vi "IVIS FRET_Load Image Data.vi"(6 "Background File Name":string="luminescent.TIF", 8 "Error In":errorcluster, 9 "# Frames":i32, 10 "Data Folder Root Name":string, 11 "Root Folder":path) -> (0 "Error Out":errorcluster, 1 "[DA Images]":T1[](array[typedef]), 2 "[AA Images]":T1[](array[typedef]), 3 "[DD Images]":T1[](array[typedef]), 4 "Time Stamps":i64[](array[numeric]), 5 "Y Resolution":i32, 7 "X Resolution":i32)   [LabVIEW 2021]
uses:
  <vilib>/vision/Image Controls.llb/IMAQ Image.ctl
  <vilib>/vision/NI_Vision_Development_Module.lvlib
panel:
  out "Same Sizes":bool
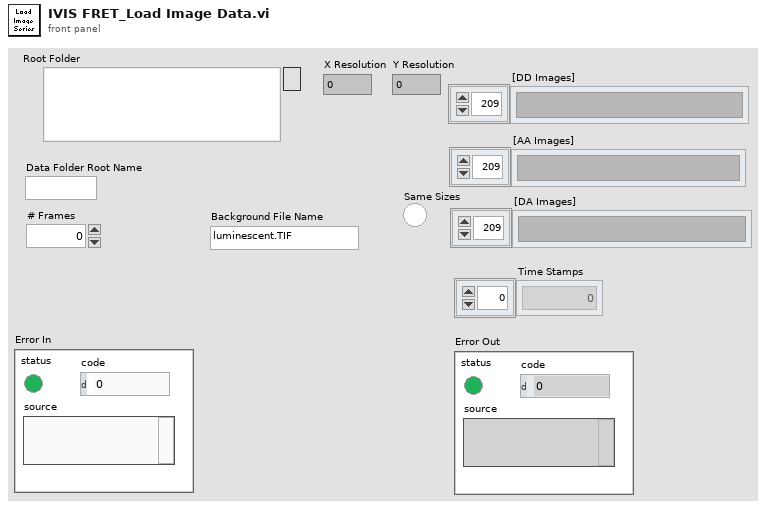
[diagram p1: front panel]
types:
  T1 = typedef "IMAQ Image.ctl" = refnum<image>
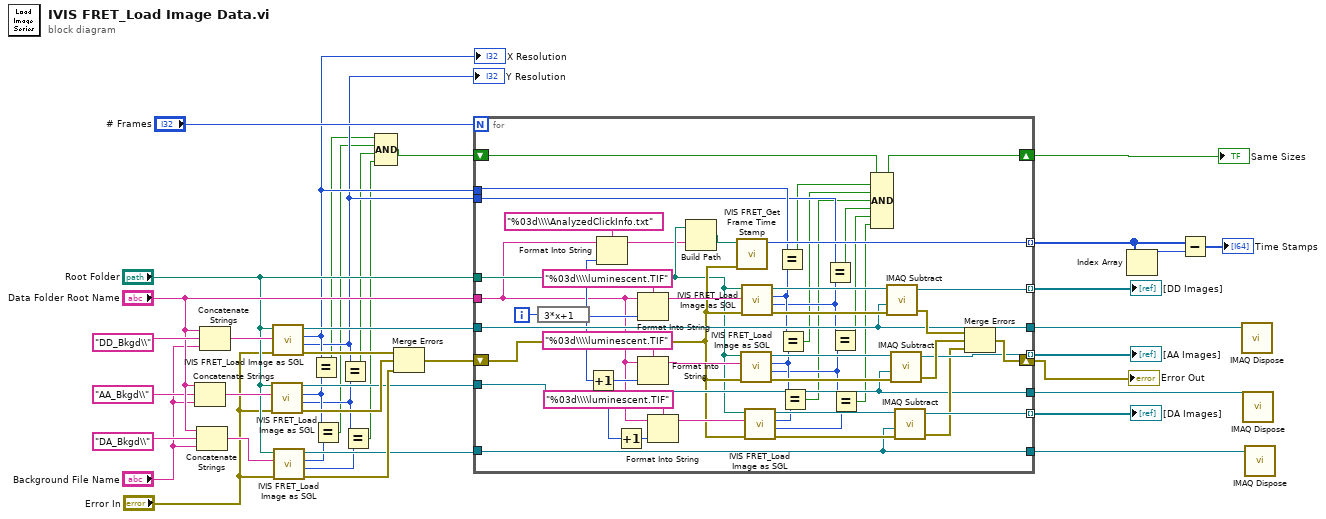
[diagram p0: block diagram]
diagram:
  n1 = Concatenate Strings("Data Folder Root Name", "AA_Bkgd\\" ("format string"), "Background File Name") -> (w27:string)
  n2 = Concatenate Strings("Data Folder Root Name", "DA_Bkgd\\" ("format string"), "Background File Name") -> (w25:string)
  n3 = Concatenate Strings("Data Folder Root Name", "DD_Bkgd\\" ("format string"), "Background File Name") -> (w35:string)
  n4 = call "IVIS FRET_Load Image as SGL.vi"("error in"="Error In", "Image File Name"=w27, "Root Folder"="Root Folder") -> ("error out"=w23:errorcluster, "Y Resolution"=w8:i32, "X Resolution"=w11:i32, "Background Image"=w20:T1)  [unwired: 5 in]
  n5 = call "IVIS FRET_Load Image as SGL.vi"("error in"="Error In", "Image File Name"=w35, "Root Folder"="Root Folder") -> ("error out"=w31:errorcluster, "Y Resolution"=w9:i32, "X Resolution"=w12:i32, "Background Image"=w29:T1)  [unwired: 5 in]
  "X Resolution" <- w12
  "Y Resolution" <- w9
  n6 = call "IVIS FRET_Load Image as SGL.vi"("error in"="Error In", "Image File Name"=w25, "Root Folder"="Root Folder") -> ("error out"=w22:errorcluster, "Y Resolution"=w7:i32, "X Resolution"=w10:i32, "Background Image"=w21:T1)  [unwired: 5 in]
  n7 = Equal?(x=w12, y=w11) -> (x = y?=w6:bool)
  n8 = Equal?(x=w11, y=w10) -> (x = y?=w5:bool)
  n9 = Equal?(x=w9, y=w8) -> (x = y?=w4:bool)
  n10 = Equal?(x=w8, y=w7) -> (x = y?=w3:bool)
  n11 = Compound Arithmetic op=AND(w6, w5, w4, w3) -> (w2:bool)
  n12 = Merge Errors(w31, w23, w22) -> (w28:errorcluster)
  n13 = for {
    N: "# Frames" -> [_]
    tunnel: "Root Folder" -> [w61]
    tunnel: "Data Folder Root Name" -> [w57]
    shift-right: [w86] -> w30
    shift-left: w28 -> [w62]
    tunnel: [w82] -> w39 mode=indexing
    tunnel: [w78] -> w37 mode=indexing
    tunnel: [w79] -> w38 mode=indexing
    tunnel: w29 -> [w70]
    tunnel: w21 -> [w65]
    tunnel: w20 -> [w69]
    tunnel: [w70] -> w19
    tunnel: [w69] -> w18
    tunnel: [w65] -> w17
    tunnel: [w58] -> w15 mode=indexing
    tunnel: w12 -> [w56]
    tunnel: w9 -> [w52]
    shift-right: [w41] -> w1
    shift-left: w2 -> [w42]
    i -> [w88]
    n14 = expression code="3*x+1"(w88) -> (w64:i32)
    n15 = Increment(x=w64) -> (x+1=w83:i32)
    n16 = Format Into String(format string="%03d\\\\AnalyzedClickInfo.txt", initial string=w57, w64) -> (resulting string=w60:string)  [unwired: 1 in, 1 out]
    n17 = Increment(x=w83) -> (x+1=w85:i32)
    n18 = Format Into String(format string="%03d\\\\luminescent.TIF", initial string=w57, w64) -> (resulting string=w68:string)  [unwired: 1 in, 1 out]
    n19 = Format Into String(format string="%03d\\\\luminescent.TIF", initial string=w57, w83) -> (resulting string=w67:string)  [unwired: 1 in, 1 out]
    n20 = Format Into String(format string="%03d\\\\luminescent.TIF", initial string=w57, w85) -> (resulting string=w66:string)  [unwired: 1 in, 1 out]
    n21 = Build Path(base path=w61, name or relative path=w60) -> (appended path=w59:path)
    n22 = call "IVIS FRET_Get Frame Time Stamp.vi"("error in (no error)"=w62, "File Path"=w59) -> ("Time Stamp"=w58:i64)  [unwired: 8 in, 1 out]
    n23 = call "IVIS FRET_Load Image as SGL.vi"("error in"=w62, "Image File Name"=w67, "Root Folder"=w61) -> ("error out"=w73:errorcluster, "Y Resolution"=w49:i32, "X Resolution"=w54:i32, "Background Image"=w74:T1)  [unwired: 5 in]
    n24 = call "IVIS FRET_Load Image as SGL.vi"("error in"=w62, "Image File Name"=w68, "Root Folder"=w61) -> ("error out"=w75:errorcluster, "Y Resolution"=w51:i32, "X Resolution"=w55:i32, "Background Image"=w76:T1)  [unwired: 5 in]
    n25 = call "IVIS FRET_Load Image as SGL.vi"("error in"=w62, "Image File Name"=w66, "Root Folder"=w61) -> ("error out"=w71:errorcluster, "Y Resolution"=w50:i32, "X Resolution"=w53:i32, "Background Image"=w72:T1)  [unwired: 5 in]
    n26 = Equal?(x=w56, y=w55) -> (x = y?=w48:bool)
    n27 = Equal?(x=w55, y=w54) -> (x = y?=w47:bool)
    n28 = Equal?(x=w54, y=w53) -> (x = y?=w46:bool)
    n29 = Equal?(x=w52, y=w51) -> (x = y?=w45:bool)
    n30 = Equal?(x=w51, y=w49) -> (x = y?=w44:bool)
    n31 = Equal?(x=w49, y=w50) -> (x = y?=w43:bool)
    n32 = Compound Arithmetic op=AND(w42, w48, w47, w46, w45, w44, w43) -> (w41:bool)
    n33 = call "IMAQ Subtract"("Image Src A"=w76, "Image Src B"=w70, "error in (no error)"=w75) -> ("Image Dst Out"=w82:T1, "error out"=w81:errorcluster)  [unwired: 4 in]
    n34 = call "IMAQ Subtract"("Image Src A"=w74, "Image Src B"=w69, "error in (no error)"=w73) -> ("Image Dst Out"=w79:T1, "error out"=w80:errorcluster)  [unwired: 4 in]
    n35 = call "IMAQ Subtract"("Image Src A"=w72, "Image Src B"=w65, "error in (no error)"=w71) -> ("Image Dst Out"=w78:T1, "error out"=w77:errorcluster)  [unwired: 4 in]
    n36 = Merge Errors(w81, w80, w77) -> (w86:errorcluster)
  }
  "Error Out" <- w30
  "[DD Images]" <- w39
  "[AA Images]" <- w38
  "[DA Images]" <- w37
  "Same Sizes" <- w1
  n37 = Index Array(array=w15) -> (element=w14:i64)  [unwired: 1 in]
  n38 = Subtract(x=w15, y=w14) -> (x-y=→"Time Stamps":i64[])
  n39 = call "IMAQ Dispose"("Image"=w19) -> ()  [unwired: 5 in, 1 out]
  n40 = call "IMAQ Dispose"("Image"=w18) -> ()  [unwired: 5 in, 1 out]
  n41 = call "IMAQ Dispose"("Image"=w17) -> ()  [unwired: 5 in, 1 out]
